vi "PH_Beamline.color fs-FE BL.vi"(0 "i ref in":refnum<vi>, 5 "error in (no error)":errorcluster) -> (14 "i ref out":refnum<vi>, 15 "Color State fs FE before Switch":i32, 16 "Color State Exit fs-FE":i32, 19 "error out":errorcluster)   [LabVIEW 2014, in "PH_Beamline.lvlib"]
doc: "This VI colors the fs-Frontend beamline elements."
uses:
  PH_Beamline.lvlib
  PH_SystemInformation/PH_SystemInformationEnabling State.ctl
  PH_StatusHandler/PH_StatusHandler.Status.ctl
  PH_Common/PH_Common.lvlib
  PH_SystemInformation/PH_SystemInformation.lvlib
  PH_BL-Master/PH_BL-Master.lvlib
  PH_StatusHandler/PH_StatusHandler.lvlib
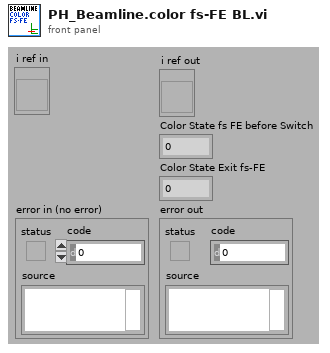
[diagram p1: front panel]
types:
  T1 = enum16{"Laser", "PreAmp", "MainAmp", "Exp 1", "Exp 2", "Exp 3", "Exp 4"}
  T2 = typedef "PH_StatusHandler.lvlib/PH_StatusHandler.Status.ctl" = i16
  T3 = typedef "PH_SystemInformation.lvlib/PH_SystemInformationEnabling State.ctl" = i32
  T4 = typedef "PH_Beamline.lvlib/PH_Beamline.i attribute.ctl" = cluster{"GUI Refs":cluster{"PA ok":refnum<vi>, "MA ok":refnum<vi>, "fs FE ok":refnum<vi>, "ns FE ok":refnum<vi>, "PA ED ok":refnum<vi>, "MAS ok":refnum<vi>, "Booster ok":refnum<vi>, "Mirrortower ok":refnum<vi>, "In.-Box ok":refnum<vi>, "Compressor ok":refnum<vi>, "Experiment LB ok":refnum<vi>, "Experiment LL ok":refnum<vi>, "PHELIX_Beckhoff_Watchdog":refnum<vi>, "Shutters closed":refnum<vi>, "uOPA ok":refnum<vi>, "Vacuum no shotcond Comp LB":refnum<vi>}, "Refs BL MA":refnum<vi>[], "Refs BL MA-IB":refnum<vi>[], "Refs BL fs":refnum<vi>[], "Refs BL PA ED":refnum<vi>[], "Refs BL MAS":refnum<vi>[], "Refs BL Boo":refnum<vi>[], "Refs BL ns":refnum<vi>[], "Refs BL Mirrortower":refnum<vi>[], "Refs BL Compressor":refnum<vi>[], "Refs BL Exp LB":refnum<vi>[], "Radiation Safety":cluster{"Exp Laserbay":cluster{"Ref Op Mode":refnum<vi>, "Ref Laserbay evacuated":refnum<vi>, "Tagname LB evacuated":string, "Shot Mode":T5, "Laserbay evacuated?":i32, "Tagname HV room locked":string, "HV room locked?":i32, "Ref HV room locked":refnum<vi>, "Tagname bridged?":string, "Ref Bridge":refnum<vi>, "I<1E18W/cm²":bool}, "Exp Laserlab":cluster{"Ref Op Mode":refnum<vi>, "Ref Laserlab evacuated":refnum<vi>, "Tagname LL evacuated":string, "Shot Mode":T5, "Laserlab evacuated?":i32, "Tagname bridged?":string, "Ref Bridge":refnum<vi>, "I<1E18W/cm²":bool}}, "Refs BL LL":refnum<vi>[], "PP Igni Heating GUI Refs":refnum<vi>[], "PP Igni Heating Tagnames ":string[], "Refs BL PA":cluster{"undelayed Line before Shutter":refnum<vi>[], "undelayed Line after Shutter":refnum<vi>[], "before Bypass":refnum<vi>[], "delayed Line before Shutter":refnum<vi>[], "delayed Line after Shutter":refnum<vi>[], "before Shutter Input":refnum<vi>[], "after Shutter Input":refnum<vi>[], "Bypass":refnum<vi>[], "before Shutter Exit":refnum<vi>[], "after Shutter Exit":refnum<vi>[], "to MA":refnum<vi>[], "to Lab":refnum<vi>[]}, "BL":cluster{"YLF_BL_Status":i32, "fs_BL_Status":i32, "fs_YLF_BL_Status":i32, "ns_BL_Status":i32, "PA_Input_BL_Status":i32, "PA_UnDelay_BL_Status":i32, "PA_Delay_BL_Status":i32, "PA_BL_Status":i32, "PA_Bypass_BL_Status":i32, "PA_Exit_BL_Status":i32, "PA_LL_BL_Status":i32, "LL_BL_Status":i32, "PA_MA_BL_Status":i32, "MA_Exit_BL_Status":i32, "MA_Z6_BL_Status":i32, "Z6_BL_Status":i32, "MA_LB_BL_Status":i32, "LB_TB2_BL_Status":i32, "PA_before_Bypass_BL_Status":i32, "LB_TB3_BL_Status":i32}, "State Subsystems":cluster{"PA":bool, "MA":bool, "ns FE":bool, "fs FE":bool, "PA ED":bool, "In.-Box":bool, "MAS":bool, "Booster":bool, "Mirrortower":bool, "Compressor":bool, "Experiment LB":bool, "Experiment LL":bool, "uOPA":bool}, "Status Subscriber Information":T6, "Refs BL uOPA":refnum<vi>[], "PA_Input_2_Beam_6PWpGUI not linked?":bool, "PA_Input_Delay_6PGUI not linked?":bool, "Settings":T9}
  T5 = typedef "PH_Beamline.lvlib/PH_Beamline.Operation Mode.ctl" = i32
  T6 = typedef "PH_Beamline.lvlib/PH_Beamline.Status Subscriber Information.ctl" = cluster{"fs Swich YLF":T7, "fs Exit Shutter":T7, "ns Exit Shutter":T7, "PA Input Shutter":T7, "PA PC WP":T7, "PA PC WP 2":T7, "PA Bypass In":T7, "PA Bypass Out":T7, "PA CH 1":T7, "PA delayed":T7, "PA non delayed":T7, "PA Exit Shutter":T7, "PA Switch Lab":T7, "PA Bridge CH Input MA":T7, "MA Diffusor IB":T7, "MA IB Ready":T7, "MA CH 1":T7, "MA CH 2":T7, "MA CH 3":T7, "MA CH 4":T7, "MA Shutter Align Cam":T7, "MA Position MM5":T7, "Calorimeter Switch":T7, "BL Z6 CH 9":T7, "BL Z6 Beamdump":T7, "BL Z6 Shutter":T7, "COS Sensitivity Switch":T7, "Exp LB Shutter":T7, "Exp LB TB 2":T7, "Exp LB TB 3":T7, "PA LL Input CH":T7, "PA LL Output CH":T7, "LL Comp Input Shutter":T7, "LL Comp Output Shutter":T7, "LL Comp FF Shutter":T7, "Exp LL Shutter":T7, "MA IM In IB":T7, "MA IM Out IB":T7, "MA DB In IB":T7, "MA DB Out IB":T7, "Exp LB Shutter Interlock":T7, "Exp LL Shutter Interlock":T7, "MM1 Force Sensor":T7}
  T7 = typedef "PH_BL-Master.lvlib/PH_BL-Master.Status Subscriber Information.ctl" = cluster{"Index of element":i32, "Attributeset":T8}
  T8 = typedef "PH_BL-Master.lvlib/PH_BL-Master.Attribute Set.ctl" = enum16{"Boolean Status Service Subscriber", "Picture Status Service Subscriber"}
  T9 = typedef "PH_Beamline_Chief.lvlib/PH_Beamline_Chief.Settings.ctl" = cluster{"PA Doublepass Mode":bool, "Compressor Vaccuum LB not relevant":bool, "Windowshutter TB2 not relevant":bool, "Windowshutter TB3 not relevant":bool}
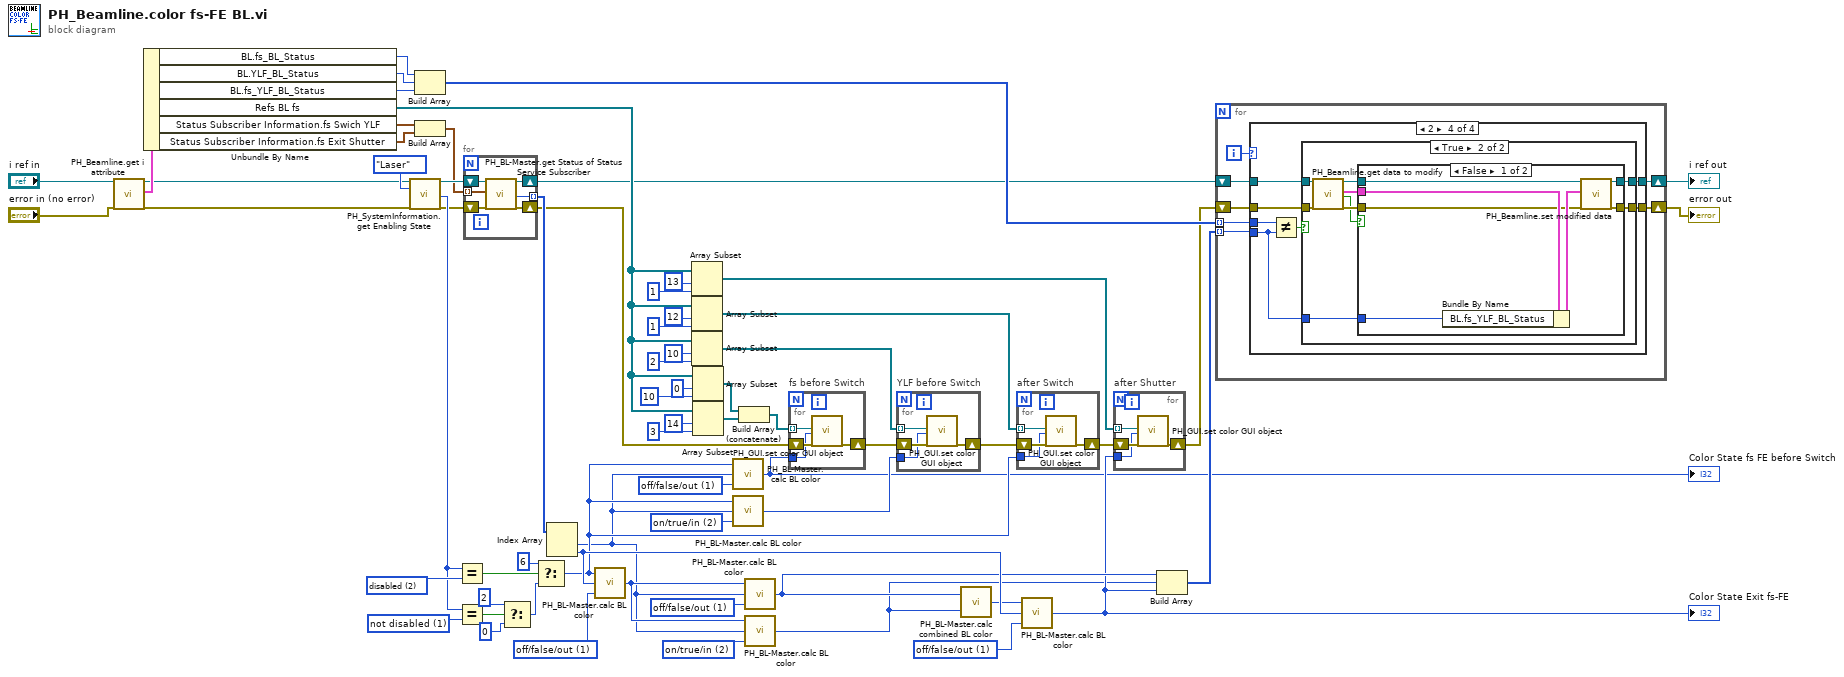
[diagram p0: block diagram]
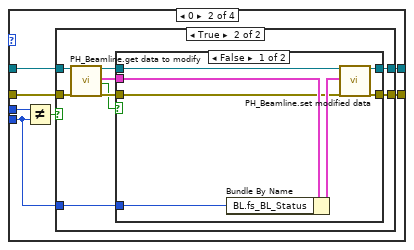
[diagram p3: hidden frame]
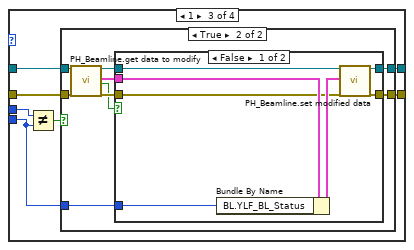
[diagram p6: hidden frame]
diagram:
  w16 = T2 2 items=["no info", "off/false/out", "on/true/in", "Failure", "Alarm", "Status 1", "Status 2", "Status 3"] ("State for \"2\" (on) of ABLE (off/false/out)")
  w17 = T2 1 items=["no info", "off/false/out", "on/true/in", "Failure", "Alarm", "Status 1", "Status 2", "Status 3"] ("State for \"2\" (on) of ABLE (off/false/out)")
  w31 = T2 1 items=["no info", "off/false/out", "on/true/in", "Failure", "Alarm", "Status 1", "Status 2", "Status 3"] ("State for \"2\" (on) of ABLE (off/false/out)")
  w33 = T2 2 items=["no info", "off/false/out", "on/true/in", "Failure", "Alarm", "Status 1", "Status 2", "Status 3"] ("State for \"2\" (on) of ABLE (off/false/out)")
  w34 = T2 1 items=["no info", "off/false/out", "on/true/in", "Failure", "Alarm", "Status 1", "Status 2", "Status 3"] ("State for \"2\" (on) of ABLE (off/false/out)")
  w35 = T2 1 items=["no info", "off/false/out", "on/true/in", "Failure", "Alarm", "Status 1", "Status 2", "Status 3"] ("State for \"2\" (on) of ABLE (off/false/out)")
  w41 = T3 2 items=["no info", "not disabled", "disabled"] ("y")
  w42 = T3 1 items=["no info", "not disabled", "disabled"] ("y")
  n1 = call "PH_Beamline.get i attribute.vi"("i ref in"="i ref in", "error in (no error)"="error in (no error)") -> ("i ref out"=w8:refnum<vi>, "i attribute"=w67:T4, "error out"=w7:errorcluster)  [unwired: 15 in]
  n2 = Unbundle By Name(w67) -> ("BL.fs_BL_Status"=w28:i32, "BL.YLF_BL_Status"=w27:i32, "BL.fs_YLF_BL_Status"=w26:i32, "Refs BL fs"=w50:refnum<vi>[], "Status Subscriber Information.fs Swich YLF"=w4:T7, "Status Subscriber Information.fs Exit Shutter"=w3:T7)
  n3 = call "PH_SystemInformation.get Enabling State.vi"("i ref in"=w8, "Wanted State"=T1."Laser", "error in (no error)"=w7) -> ("i ref out"=w30:refnum<vi>, "Enabling State"=w37:T3, "error out"=w29:errorcluster)  [unwired: 14 in]
  n4 = Build Array(w28, w27, w26) -> (w25:i32[])
  n5 = Build Array(w4, w3) -> (w2:T7[])
  n6 = Equal?(x=w37, y=w41) -> (x = y?=w45:bool)
  n7 = Equal?(x=w37, y=w42) -> (x = y?=w43:bool)
  n8 = for {
    tunnel: w2 -> [w73] mode=indexing
    shift-right: [w71] -> w5
    shift-left: w30 -> [w72]
    shift-right: [w69] -> w6
    shift-left: w29 -> [w70]
    tunnel: [w68] -> w46 mode=indexing
    n9 = call "PH_BL-Master.get Status of Status Service Subscriber.vi"("i ref in"=w72, "Wanted Status Subscriber Information"=w73, "error in (no error)"=w70) -> ("i ref out"=w71:refnum<vi>, "Status"=w68:T2, "error out"=w69:errorcluster)  [unwired: 11 in, 3 out]
  }
  n10 = Select(t=2 ("State before ABLE"), s=w43, f=0) -> (s? t:f=w39:i32)
  n11 = Select(t=6 ("State before ABLE"), s=w45, f=w39) -> (s? t:f=w15:i32)
  n12 = Index Array(array=w46) -> (element #1=w14:T2, element #2=w32:T2)  [unwired: 2 in]
  n13 = call "PH_BL-Master.calc BL color.vi"("State for \"2\" (on) of ABLE (off/false/out)"=w35, "State ABLE"=w32, "State before ABLE"=w15) -> ("State after ABLE"=w36:i32)
  n14 = Array Subset(array=w50, index=13, length=1) -> (w53:refnum<vi>[])
  n15 = Array Subset(array=w50, index=12, length=1) -> (w57:refnum<vi>[])
  n16 = Array Subset(array=w50, index=10, length=2) -> (w60:refnum<vi>[])
  n17 = Array Subset(array=w50, index=0, length=10) -> (w48:refnum<vi>[])
  n18 = Array Subset(array=w50, index=14, length=3) -> (w49:refnum<vi>[])
  n19 = call "PH_BL-Master.calc BL color.vi"("State for \"2\" (on) of ABLE (off/false/out)"=w17, "State ABLE"=w14, "State before ABLE"=w15) -> ("State after ABLE"=w1:i32)
  "Color State fs FE before Switch" <- w1
  n20 = call "PH_BL-Master.calc BL color.vi"("State for \"2\" (on) of ABLE (off/false/out)"=w16, "State ABLE"=w14, "State before ABLE"=w15) -> ("State after ABLE"=w13:i32)
  n21 = Build Array (concatenate)(w48, w49) -> (w47:refnum<vi>[])
  n22 = call "PH_BL-Master.calc BL color.vi"("State for \"2\" (on) of ABLE (off/false/out)"=w34, "State ABLE"=w14, "State before ABLE"=w36) -> ("State after ABLE"=w24:i32)
  n23 = call "PH_BL-Master.calc BL color.vi"("State for \"2\" (on) of ABLE (off/false/out)"=w33, "State ABLE"=w14, "State before ABLE"=w36) -> ("State after ABLE"=w12:i32)
  n24 = for "fs before Switch" {
    tunnel: w47 -> [w77] mode=indexing
    shift-right: [w75] -> w59
    shift-left: w6 -> [w76]
    tunnel: w1 -> [w74]
    n25 = call "PH_GUI.set color GUI object.vi"("GUI object Ref"=w77, "State"=w74, "error in (no error)"=w76) -> ("error out"=w75:errorcluster)  [unwired: 16 in]
  }
  n26 = for "YLF before Switch" {
    tunnel: w60 -> [w81] mode=indexing
    shift-right: [w79] -> w58
    shift-left: w59 -> [w80]
    tunnel: w13 -> [w78]
    n27 = call "PH_GUI.set color GUI object.vi"("GUI object Ref"=w81, "State"=w78, "error in (no error)"=w80) -> ("error out"=w79:errorcluster)  [unwired: 16 in]
  }
  n28 = call "PH_BL-Master.calc combined BL color.vi"("Color State BL 2"=w12, "Color State BL 1"=w24) -> ("Color State combined BL"=w18:i32)
  n29 = for "after Switch" {
    tunnel: w57 -> [w85] mode=indexing
    shift-right: [w83] -> w56
    shift-left: w58 -> [w84]
    tunnel: w15 -> [w82]
    n30 = call "PH_GUI.set color GUI object.vi"("GUI object Ref"=w85, "State"=w82, "error in (no error)"=w84) -> ("error out"=w83:errorcluster)  [unwired: 16 in]
  }
  n31 = call "PH_BL-Master.calc BL color.vi"("State for \"2\" (on) of ABLE (off/false/out)"=w31, "State ABLE"=w32, "State before ABLE"=w18) -> ("State after ABLE"=w23:i32)
  "Color State Exit fs-FE" <- w23
  n32 = for "after Shutter" {
    tunnel: w53 -> [w89] mode=indexing
    shift-right: [w87] -> w19
    shift-left: w56 -> [w88]
    tunnel: w23 -> [w86]
    n33 = call "PH_GUI.set color GUI object.vi"("GUI object Ref"=w89, "State"=w86, "error in (no error)"=w88) -> ("error out"=w87:errorcluster)  [unwired: 16 in]
  }
  n34 = Build Array(w24, w12, w23) -> (w22:i32[])
  n35 = for {
    shift-right: [w95] -> w21
    shift-left: w5 -> [w93]
    shift-right: [w94] -> w20
    shift-left: w19 -> [w92]
    tunnel: w25 -> [w91] mode=indexing
    tunnel: w22 -> [w90] mode=indexing
    i -> [w96]
    n36 = case shown="2" w96 {
      tunnel: [w97 w104 w131 w158] -> w94
      tunnel: w92 -> [w97 w103 w130 w157]
      tunnel: [w98 w102 w129 w156] -> w95
      tunnel: w93 -> [w98 w101 w128 w155]
      tunnel: w90 -> [_ w100 w127 w154]
      tunnel: w91 -> [_ w99 w126 w153]
      frame Default {
      }
      frame 0 {
        n37 = Not Equal?(x=w99, y=w100) -> (x != y?=w105:bool)
        n38 = case shown="True" w105 {
          tunnel: w101 -> [w107 w112]
          tunnel: [w107 w111] -> w102
          tunnel: w103 -> [w106 w110]
          tunnel: [w106 w109] -> w104
          tunnel: w100 -> [_ w108]
          frame False {
          }
          frame True {
            n39 = call "PH_Beamline.get data to modify.vi"("i ref in"=w112, "error in (no error)"=w110) -> ("i ref out"=w115:refnum<vi>, "i attribute"=w113:T4, "timed out"=w114:bool, "error out"=w116:errorcluster)  [unwired: 14 in]
            n40 = case shown="False" w114 {
              tunnel: w116 -> [w117 w124]
              tunnel: w115 -> [w123 w125]
              tunnel: [w122 w124] -> w109
              tunnel: [w121 w125] -> w111
              tunnel: w113 -> [w118 _]
              tunnel: w108 -> [w119 _]
              frame False {
                n41 = Bundle By Name(cluster=w118, "BL.fs_BL_Status"=w119) -> (w120:T4)
                n42 = call "PH_Beamline.set modified data.vi"("i ref in"=w123, "i attribute"=w120, "error in (no error)"=w117) -> ("i ref out"=w121:refnum<vi>, "error out"=w122:errorcluster)  [unwired: 15 in]
              }
              frame True {
              }
            }
          }
        }
      }
      frame 1 {
        n43 = Not Equal?(x=w126, y=w127) -> (x != y?=w132:bool)
        n44 = case shown="True" w132 {
          tunnel: w128 -> [w134 w139]
          tunnel: [w134 w138] -> w129
          tunnel: w130 -> [w133 w137]
          tunnel: [w133 w136] -> w131
          tunnel: w127 -> [_ w135]
          frame False {
          }
          frame True {
            n45 = call "PH_Beamline.get data to modify.vi"("i ref in"=w139, "error in (no error)"=w137) -> ("i ref out"=w142:refnum<vi>, "i attribute"=w140:T4, "timed out"=w141:bool, "error out"=w143:errorcluster)  [unwired: 14 in]
            n46 = case shown="False" w141 {
              tunnel: w143 -> [w144 w151]
              tunnel: w142 -> [w150 w152]
              tunnel: [w149 w151] -> w136
              tunnel: [w148 w152] -> w138
              tunnel: w140 -> [w145 _]
              tunnel: w135 -> [w146 _]
              frame False {
                n47 = Bundle By Name(cluster=w145, "BL.YLF_BL_Status"=w146) -> (w147:T4)
                n48 = call "PH_Beamline.set modified data.vi"("i ref in"=w150, "i attribute"=w147, "error in (no error)"=w144) -> ("i ref out"=w148:refnum<vi>, "error out"=w149:errorcluster)  [unwired: 15 in]
              }
              frame True {
              }
            }
          }
        }
      }
      frame 2 {
        n49 = Not Equal?(x=w153, y=w154) -> (x != y?=w159:bool)
        n50 = case shown="True" w159 {
          tunnel: w155 -> [w161 w166]
          tunnel: [w161 w165] -> w156
          tunnel: w157 -> [w160 w164]
          tunnel: [w160 w163] -> w158
          tunnel: w154 -> [_ w162]
          frame False {
          }
          frame True {
            n51 = call "PH_Beamline.get data to modify.vi"("i ref in"=w166, "error in (no error)"=w164) -> ("i ref out"=w169:refnum<vi>, "i attribute"=w167:T4, "timed out"=w168:bool, "error out"=w170:errorcluster)  [unwired: 14 in]
            n52 = case shown="False" w168 {
              tunnel: w170 -> [w171 w178]
              tunnel: w169 -> [w177 w179]
              tunnel: [w176 w178] -> w163
              tunnel: [w175 w179] -> w165
              tunnel: w167 -> [w172 _]
              tunnel: w162 -> [w173 _]
              frame False {
                n53 = Bundle By Name(cluster=w172, "BL.fs_YLF_BL_Status"=w173) -> (w174:T4)
                n54 = call "PH_Beamline.set modified data.vi"("i ref in"=w177, "i attribute"=w174, "error in (no error)"=w171) -> ("i ref out"=w175:refnum<vi>, "error out"=w176:errorcluster)  [unwired: 15 in]
              }
              frame True {
              }
            }
          }
        }
      }
    }
  }
  "error out" <- w20
  "i ref out" <- w21
